vi "Query Marker.vi"(8 "error in (no error)":errorcluster, 10 "Active Marker (1: Marker 1)":i32(ring)=1 items=["Marker 1"=1, "Marker 2"=2, "Marker 3"=3, "Marker 4"=4, "Marker 5"=5, "Marker 6"=6], 11 "VISA resource name":refnum<visa-resource-name>) -> (0 "error out":errorcluster, 2 "Y Value":dbl, 3 "VISA resource name out":refnum<visa-resource-name>)   [LabVIEW 2022 SP3, in "Agilent N934X Series.lvlib"]
doc: "Returns the x-position and amplitude of a specified marker."
uses:
  <instrlib>/Agilent N934X Series/Agilent N934X Series.lvlib
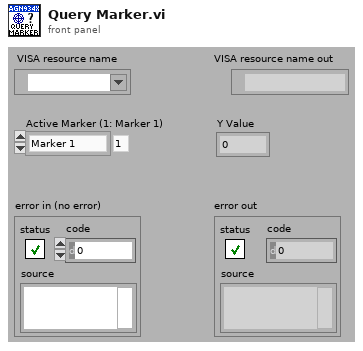
[diagram p1: front panel]
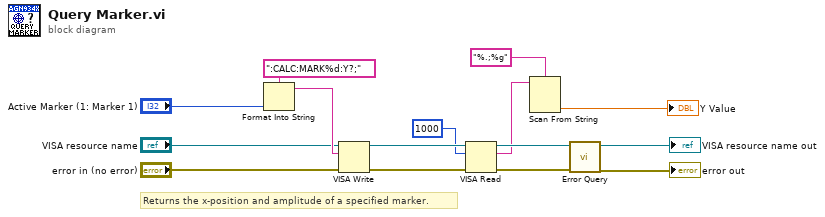
[diagram p0: block diagram]
diagram:
  # "Returns the x-position and amplitude of a specified marker."
  n1 = Format Into String(format string=":CALC:MARK%d:Y?;", "Active Marker (1: Marker 1)") -> (resulting string=w13:string)  [unwired: 2 in, 1 out]
  n2 = VISA Write(VISA resource name="VISA resource name", write buffer=w13, error in (no error)="error in (no error)") -> (VISA resource name out=w8:refnum<visa-resource-name>, error out=w7:errorcluster)  [unwired: 1 out]
  n3 = VISA Read(VISA resource name=w8, byte count=u32 1000, error in (no error)=w7) -> (VISA resource name out=w6:refnum<visa-resource-name>, read buffer=w1:string, error out=w5:errorcluster)  [unwired: 1 out]
  n4 = Scan From String(format string="%.;%g", input string=w1) -> (output 1=→"Y Value":dbl)  [unwired: 3 in, 3 out]
  n5 = call <instrlib>:"Error Query.vi"("error in (no error)"=w5, "VISA resource name"=w6) -> ("error out"=→"error out":errorcluster, "VISA resource name out"=→"VISA resource name out":refnum<visa-resource-name>)  [unwired: 6 in, 2 out]
